vi "20220114 main.vi"() -> ()   [LabVIEW 2019]
uses:
  subVI/move/position cluster.ctl
  subVI/move/move array.ctl
  subVI/arduino/Servo/servo option.ctl
  <vilib>/myRIO/Common/Instrument Driver Framework/myRIO v1.0/UART/vis/myRIO v1.0 Close UART.vi
  <vilib>/myRIO/Common/Instrument Driver Framework/Utilities/vis/FPGA Ref Manager.vi
  <vilib>/myRIO/Common/Instrument Driver Framework/myRIO v1.0/myRIO v1.0 Reset FPGA.vi
  <vilib>/myRIO/Common/Instrument Driver Framework/myRIO v1.0/IRQ/vis/myRIO v1.0 IRQ Info FGV.vi
  <vilib>/myRIO/Common/Instrument Driver Framework/myRIO v1.0/IRQ/vis/myRIO v1.0 Timer IRQ Info FGV.vi
  <vilib>/myRIO/Common/Instrument Driver Framework/myRIO v1.0/IRQ/vis/myRIO v1.0 ISR Agent.vi
  <vilib>/myRIO/Instrument Drivers/Utilities/vis/Reset Index.vi
  <vilib>/myRIO/Common/Instrument Driver Framework/myRIO v1.0/Resource Manager/vis/myRIO v1.0 Block Write Resource Manager.vi
  <vilib>/myRIO/Instrument Drivers/Utilities/Utilities.lvlib
panel:
  out "error out":errorcluster
  in  "error in (no error)":errorcluster
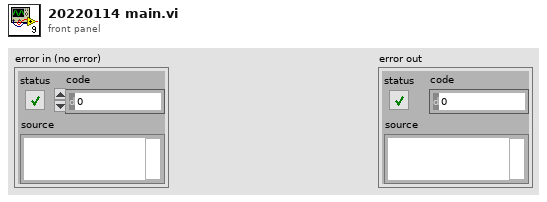
[diagram p1: front panel]
types:
  T1 = typedef "position cluster.ctl" = cluster{"X":dbl, "Y":dbl, "Angle":dbl}
  T2 = enum16{"init", "vision", "vision go to catch", "catch", "A zone to B zone", "B zone put", "goto home"}[]
  T3 = typedef "servo option.ctl" = enum8{"", "put", "catch", "vision-1", "vision-2"}
  T4 = typedef "move array.ctl" = cluster{"X":dbl, "Y":dbl}[]
  T5 = enum16{"init", "vision", "vision go to catch", "catch", "A zone to B zone", "B zone put", "goto home"}
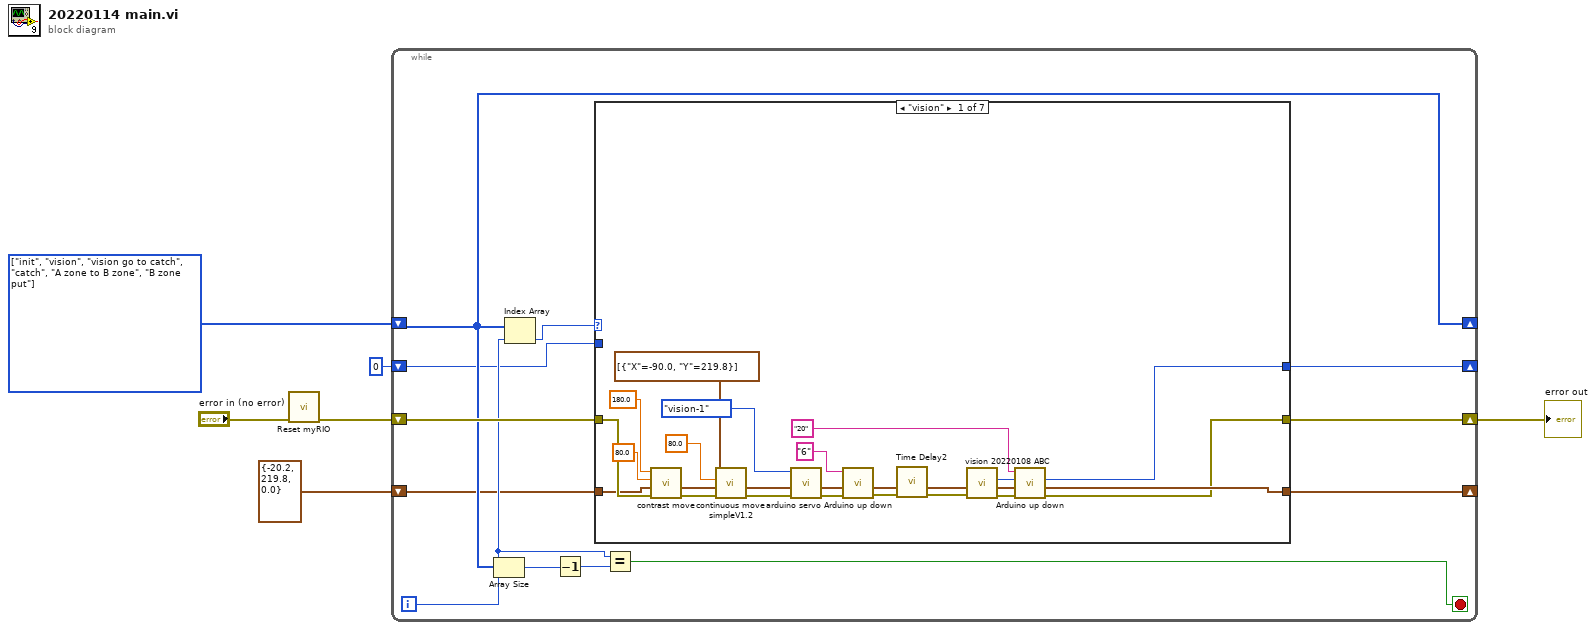
[diagram p0: block diagram]
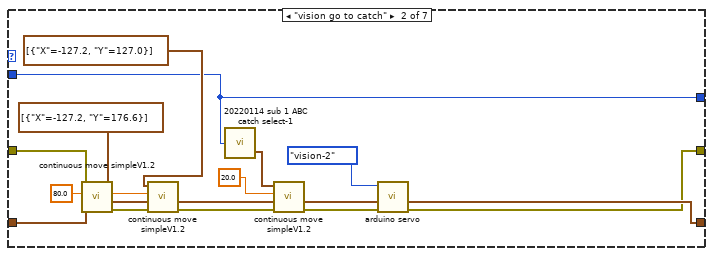
[diagram p2: hidden frame]
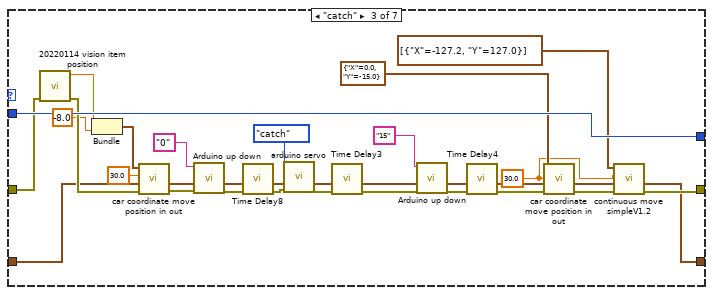
[diagram p3: hidden frame]
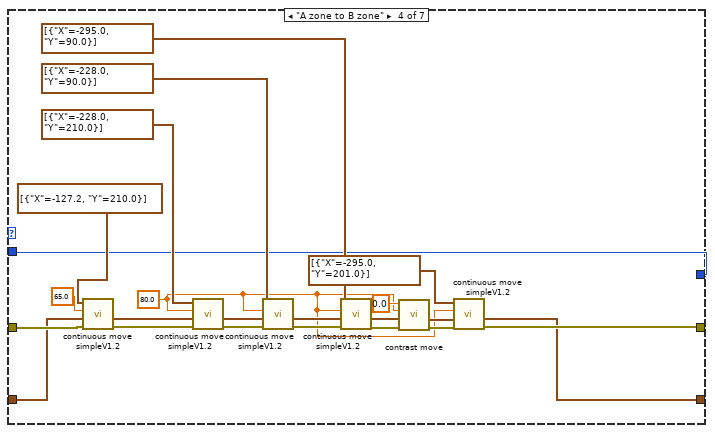
[diagram p4: hidden frame]
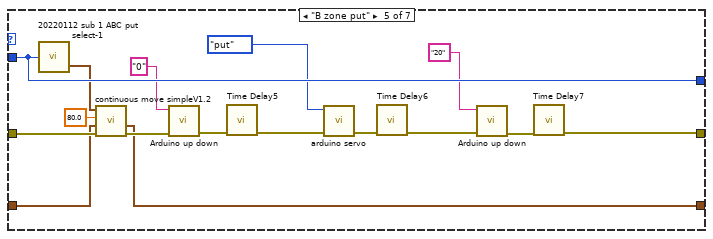
[diagram p5: hidden frame]
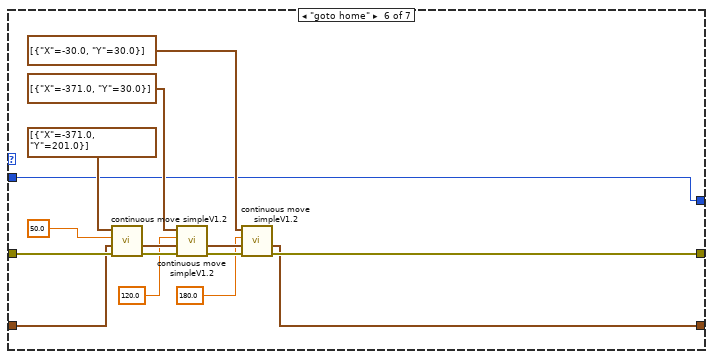
[diagram p6: hidden frame]
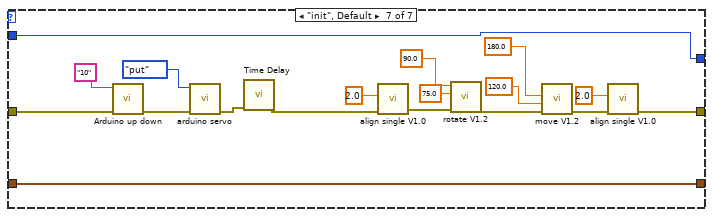
[diagram p7: hidden frame]
diagram:
  w4 = T2 [enum."init", enum."vision", enum."vision go to catch", enum."catch", enum."A zone to B zone", enum."B zone put"] items=["init", "vision", "vision go to catch", "catch", "A zone to B zone", "B zone put", "goto home"]
  n1 = call <vilib>:"Reset myRIO.vi"("error in (no error)"="error in (no error)") -> ("error out"=w1:errorcluster)  [unwired: 10 in]
  n2 = while {
    shift-right: [w17] -> w5
    shift-left: w1 -> [w18]
    shift-right: [w15] -> _
    shift-left: w4 -> [w15]
    shift-right: [w9] -> _
    shift-left: T1 {"X"=-20.2, "Y"=219.8, "Angle"=0.0} ("Position") -> [w10]
    shift-right: [w8] -> _
    shift-left: 0 ("index of wood") -> [w7]
    i -> [w13]
    stop <- w12 stop-if-true
    n3 = Array Size(array=w15) -> (size(s)=w14:i32)
    n4 = Index Array(array=w15, index=w13) -> (element=w16:T5)
    n5 = Decrement(x=w14) -> (x-1=w11:i32)
    n6 = case shown="\"vision\"" w16 {
      tunnel: w18 -> [w37 w53 w65 w102 w117 w133 w137]
      tunnel: [w19 w38 w67 w81 w103 w122 w136] -> w17
      tunnel: w10 -> [w36 w52 w62 w101 w116 w132 w135]
      tunnel: [w29 w42 w66 w80 w105 w121 w135] -> w9
      tunnel: [w22 w46 w74 w89 w118 w120 w134] -> w8
      tunnel: w7 -> [_ w46 w74 w89 w118 w120 w134]
      frame "vision" {
        n7 = call "contrast move.vi"("error in (no error)"=w37, "Position in"=w36, "speed"=80.0, "Target degree"=180.0) -> ("error out"=w33:errorcluster, "Position out"=w32:T1)  [unwired: 6 in]
        n8 = call "continuous move simpleV1.2.vi"("error in (no error)"=w33, "Position"=w32, "Speed"=80.0, "Array"=T4 [{"X"=-90.0, "Y"=219.8}]) -> ("error out"=w28:errorcluster, "Position out"=w29:T1)  [unwired: 6 in]
        n9 = call "arduino servo.vi"("error in (no error)"=w28, "Enum"=servo_option."vision-1") -> ("error out"=w26:errorcluster)  [unwired: 9 in]
        n10 = call "Arduino up down.vi"("error in (no error)"=w26, "Height"="6") -> ("error out"=w24:errorcluster)  [unwired: 9 in]
        n11 = call "Time Delay2"("error in (no error)"=w24) -> ("error out"=w23:errorcluster)  [unwired: 10 in]
        n12 = call "vision 20220108 ABC.vi"("error in"=w23) -> ("error out"=w21:errorcluster, "index of wood"=w22:i32)  [unwired: 5 in]
        n13 = call "Arduino up down.vi"("error in (no error)"=w21, "Height"="20") -> ("error out"=w19:errorcluster)  [unwired: 9 in]
      }
      frame "vision go to catch" {
        w48 = 80.0 ("Speed")
        n14 = call "continuous move simpleV1.2.vi"("error in (no error)"=w53, "Position"=w52, "Speed"=w48, "Array"=T4 [{"X"=-127.2, "Y"=176.6}]) -> ("error out"=w50:errorcluster, "Position out"=w49:T1)  [unwired: 6 in]
        n15 = call "continuous move simpleV1.2.vi"("error in (no error)"=w50, "Position"=w49, "Speed"=w48, "Array"=T4 [{"X"=-127.2, "Y"=127.0}]) -> ("error out"=w41:errorcluster, "Position out"=w45:T1)  [unwired: 6 in]
        n16 = call "20220114 sub 1 ABC catch select-1.vi"("ABC"=w46) -> ("ABC path out go catch"=w44:cluster{"X":dbl, "Y":dbl}[])  [unwired: 1 in]
        n17 = call "continuous move simpleV1.2.vi"("error in (no error)"=w41, "Position"=w45, "Speed"=20.0, "Array"=w44) -> ("error out"=w39:errorcluster, "Position out"=w42:T1)  [unwired: 6 in]
        n18 = call "arduino servo.vi"("error in (no error)"=w39, "Enum"=servo_option."vision-2") -> ("error out"=w38:errorcluster)  [unwired: 9 in]
      }
      frame "catch" {
        w68 = 30.0 ("speed")
        n19 = call "20220114 vision item position.vi"("error in"=w65) -> ("error out"=w64:errorcluster, "Numeric"=w61:dbl)  [unwired: 9 in]
        n20 = Bundle("Numeric"=w61, -8.0) -> (w59:cluster{"Numeric":dbl, dbl})  [unwired: 1 in]
        n21 = call "car coordinate move position in out.vi"("error in (no error)"=w64, "Position in"=w62, "speed"=30.0, "move"=w59) -> ("error out"=w57:errorcluster, "Position out"=w63:T1)  [unwired: 6 in]
        n22 = call "Arduino up down.vi"("error in (no error)"=w57, "Height"="0") -> ("error out"=w54:errorcluster)  [unwired: 9 in]
        n23 = call "Time Delay8"("error in (no error)"=w54) -> ("error out"=w55:errorcluster)  [unwired: 10 in]
        n24 = call "arduino servo.vi"("error in (no error)"=w55, "Enum"=servo_option."catch") -> ("error out"=w78:errorcluster)  [unwired: 9 in]
        n25 = call "Time Delay3"("error in (no error)"=w78) -> ("error out"=w77:errorcluster)  [unwired: 10 in]
        n26 = call "Arduino up down.vi"("error in (no error)"=w77, "Height"="15") -> ("error out"=w75:errorcluster)  [unwired: 9 in]
        n27 = call "Time Delay4"("error in (no error)"=w75) -> ("error out"=w73:errorcluster)  [unwired: 10 in]
        n28 = call "car coordinate move position in out.vi"("error in (no error)"=w73, "Position in"=w63, "speed"=w68, "move"=cluster{"X":dbl, "Y":dbl} {"X"=0.0, "Y"=-15.0}) -> ("error out"=w69:errorcluster, "Position out"=w70:T1)  [unwired: 6 in]
        n29 = call "continuous move simpleV1.2.vi"("error in (no error)"=w69, "Position"=w70, "Speed"=w68, "Array"=T4 [{"X"=-127.2, "Y"=127.0}]) -> ("error out"=w67:errorcluster, "Position out"=w66:T1)  [unwired: 6 in]
      }
      frame "A zone to B zone" {
        w82 = 80.0 ("Speed")
        n30 = call "continuous move simpleV1.2.vi"("error in (no error)"=w102, "Position"=w101, "Speed"=65.0, "Array"=T4 [{"X"=-127.2, "Y"=210.0}]) -> ("error out"=w91:errorcluster, "Position out"=w90:T1)  [unwired: 6 in]
        n31 = call "continuous move simpleV1.2.vi"("error in (no error)"=w91, "Position"=w90, "Speed"=w82, "Array"=T4 [{"X"=-228.0, "Y"=210.0}]) -> ("error out"=w95:errorcluster, "Position out"=w96:T1)  [unwired: 6 in]
        n32 = call "continuous move simpleV1.2.vi"("error in (no error)"=w95, "Position"=w96, "Speed"=w82, "Array"=T4 [{"X"=-228.0, "Y"=90.0}]) -> ("error out"=w94:errorcluster, "Position out"=w93:T1)  [unwired: 6 in]
        n33 = call "continuous move simpleV1.2.vi"("error in (no error)"=w94, "Position"=w93, "Speed"=w82, "Array"=T4 [{"X"=-295.0, "Y"=90.0}]) -> ("error out"=w88:errorcluster, "Position out"=w87:T1)  [unwired: 6 in]
        n34 = call "contrast move.vi"("error in (no error)"=w88, "Position in"=w87, "speed"=w82, "Target degree"=0.0) -> ("error out"=w85:errorcluster, "Position out"=w84:T1)  [unwired: 6 in]
        n35 = call "continuous move simpleV1.2.vi"("error in (no error)"=w85, "Position"=w84, "Speed"=w82, "Array"=T4 [{"X"=-295.0, "Y"=201.0}]) -> ("error out"=w81:errorcluster, "Position out"=w80:T1)  [unwired: 6 in]
      }
      frame "B zone put" {
        n36 = call "20220112 sub 1 ABC put select-1.vi"("ABC"=w118) -> ("ABC path out go catch"=w114:cluster{"X":dbl, "Y":dbl}[])  [unwired: 1 in]
        n37 = call "continuous move simpleV1.2.vi"("error in (no error)"=w117, "Position"=w116, "Speed"=80.0, "Array"=w114) -> ("error out"=w113:errorcluster, "Position out"=w105:T1)  [unwired: 6 in]
        n38 = call "Arduino up down.vi"("error in (no error)"=w113, "Height"="0") -> ("error out"=w111:errorcluster)  [unwired: 9 in]
        n39 = call "Time Delay5"("error in (no error)"=w111) -> ("error out"=w110:errorcluster)  [unwired: 10 in]
        n40 = call "arduino servo.vi"("error in (no error)"=w110, "Enum"=servo_option."put") -> ("error out"=w108:errorcluster)  [unwired: 9 in]
        n41 = call "Time Delay6"("error in (no error)"=w108) -> ("error out"=w107:errorcluster)  [unwired: 10 in]
        n42 = call "Arduino up down.vi"("error in (no error)"=w107, "Height"="20") -> ("error out"=w104:errorcluster)  [unwired: 9 in]
        n43 = call "Time Delay7"("error in (no error)"=w104) -> ("error out"=w103:errorcluster)  [unwired: 10 in]
      }
      frame "goto home" {
        n44 = call "continuous move simpleV1.2.vi"("error in (no error)"=w133, "Position"=w132, "Speed"=50.0, "Array"=T4 [{"X"=-371.0, "Y"=201.0}]) -> ("error out"=w129:errorcluster, "Position out"=w128:T1)  [unwired: 6 in]
        n45 = call "continuous move simpleV1.2.vi"("error in (no error)"=w129, "Position"=w128, "Speed"=120.0, "Array"=T4 [{"X"=-371.0, "Y"=30.0}]) -> ("error out"=w126:errorcluster, "Position out"=w125:T1)  [unwired: 6 in]
        n46 = call "continuous move simpleV1.2.vi"("error in (no error)"=w126, "Position"=w125, "Speed"=180.0, "Array"=T4 [{"X"=-30.0, "Y"=30.0}]) -> ("error out"=w122:errorcluster, "Position out"=w121:T1)  [unwired: 6 in]
      }
      frame "init", Default {
        n47 = call "Arduino up down.vi"("error in (no error)"=w137, "Height"="10") -> ("error out"=w141:errorcluster)  [unwired: 9 in]
        n48 = call "arduino servo.vi"("error in (no error)"=w141, "Enum"=enum8{"", "put", "catch"}."put") -> ("error out"=w139:errorcluster)  [unwired: 9 in]
        n49 = call "Time Delay"("error in (no error)"=w139) -> ("error out"=w138:errorcluster)  [unwired: 10 in]
        n50 = call "align single V1.0.vi"("error in (no error)"=w138, "Target (Volt)"=2.0) -> ("error out"=w150:errorcluster)  [unwired: 9 in]
        n51 = call "rotate V1.2.vi"("error in (no error)"=w150, "speed"=75.0, "degree"=90.0) -> ("error out"=w147:errorcluster)  [unwired: 8 in]
        n52 = call "move V1.2.vi"("error in (no error)"=w147, "RPM"=120.0, "Y"=180.0) -> ("error out"=w143:errorcluster)  [unwired: 8 in]
        n53 = call "align single V1.0.vi"("error in (no error)"=w143, "Target (Volt)"=2.0) -> ("error out"=w136:errorcluster)  [unwired: 9 in]
      }
    }
    n54 = Equal?(x=w13, y=w11) -> (x = y?=w12:bool)
  }
  "error out" <- w5
